vi "XBMC Send Input Action.vi"() -> ()   [LabVIEW 2013, in "LVH-XBMC.lvlib"]
doc: "This example demonstrates how to send basic input actions to a local or remote XBMC instance."
uses:
  vi.lib/LabVIEW Hacker/XBMC/LVH-XBMC.lvlib
  vi.lib/LabVIEW Hacker/XBMC/Private/Type Defs/JSON_Objects/Input_Action.ctl
panel:
  in  "Port (80)":u16=80
  in  "Stop Button":bool
  in  "Select Button":bool
  in  "Back Button":bool
  in  "Right Button":bool
  in  "Left Button":bool
  in  "Down Button":bool
  in  "Up Button":bool
  in  "Hostname / IP":string="localhost"
  in  "Username":string
  in  "Password":string
  # "XBMC Basic Input Action Example\n\nThis example demonstrates how to send basic input actions to a local or remote XBMC instance.\n\n1. Enter the Hostname or IP Address of the XBMC instance you want to control.\n     Note: The XBMC webserver must be enabled for the LabVIEW XBMC API to work. \n2. Enter the Username and Password you've assigned to the XBMC instance.\n3. Click the Run Arrow.\n4. Click the buttons on this LabVIEW front panel to send input actions to the XBMC instance."
  # "Configure"
  # "Control"
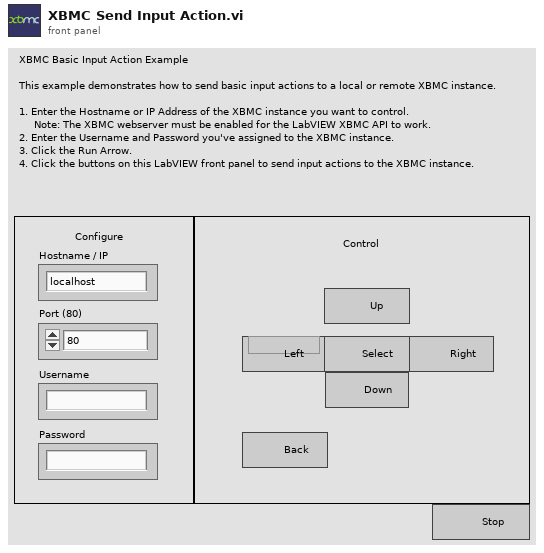
[diagram p1: front panel]
types:
  T1 = typedef "LVH-XBMC.lvlib/XBMC Ref.ctl" = cluster{"HTTP Handle":T2, "Hostname / IP":string, "jsonrpc":string}
  T2 = typedef "LabVIEWHTTPClient.lvlib/ClientHandle.ctl" = refnum<k1>
  T3 = typedef "LVH-XBMC.lvlib/Input_Action.ctl" = enum16{"left", "right", "up", "down", "pageup", "pagedown", "select", "highlight", "parentdir", "parentfolder", "back", "previousmenu", "info", "pause", "stop", "skipnext", "skipprevious", "fullscreen", "aspectratio", "stepforward", "stepback", "bigstepforward", "bigstepback", "chapterorbigstepforward", "chapterorbigstepback", "osd", "showsubtitles", "nextsubtitle", "codecinfo", "nextpicture", "previouspicture", "zoomout", "zoomin", "playlist", "queue", "zoomnormal", "zoomlevel1", "zoomlevel2", "zoomlevel3", "zoomlevel4", "zoomlevel5", "zoomlevel6", "zoomlevel7", "zoomlevel8", "zoomlevel9", "nextcalibration", "resetcalibration", "analogmove", "rotate", "rotateccw", "close", "subtitledelayminus", "subtitledelay", "subtitledelayplus", "audiodelayminus", "audiodelay", "audiodelayplus", "subtitleshiftup", "subtitleshiftdown", "subtitlealign", "audionextlanguage", "verticalshiftup", "verticalshiftdown", "nextresolution", "audiotoggledigital", "number0", "number1", "number2", "number3", "number4", "number5", "number6", "number7", "number8", "number9", "osdleft", "osdright", "osdup", "osddown", "osdselect", "osdvalueplus", "osdvalueminus", "smallstepback", "fastforward", "rewind", "play", "playpause", "switchplayer", "delete", "copy", "move", "mplayerosd", "hidesubmenu", "screenshot", "rename", "togglewatched", "scanitem", "reloadkeymaps", "volumeup", "volumedown", "mute", "backspace", "scrollup", "scrolldown", "analogfastforward", "analogrewind", "moveitemup", "moveitemdown", "contextmenu", "shift", "symbols", "cursorleft", "cursorright", "showtime", "analogseekforward", "analogseekback", "showpreset", "presetlist", "nextpreset", "previouspreset", "lockpreset", "randompreset", "increasevisrating", "decreasevisrating", "showvideomenu", "enter", "increaserating", "decreaserating", "togglefullscreen", "nextscene", "previousscene", "nextletter", "prevletter", "jumpsms2", "jumpsms3", "jumpsms4", "jumpsms5", "jumpsms6", "jumpsms7", "jumpsms8", "jumpsms9", "filter", "filterclear", "filtersms2", "filtersms3", "filtersms4", "filtersms5", "filtersms6", "filtersms7", "filtersms8", "filtersms9", "firstpage", "lastpage", "guiprofile", "red", "green", "yellow", "blue", "increasepar", "decreasepar", "volampup", "volampdown", "createbookmark", "createepisodebookmark", "settingsreset", "settingslevelchange", "stereomode", "nextstereomode", "previousstereomode", "togglestereomode", "stereomodetomono", "channelup", "channeldown", "previouschannelgroup", "nextchannelgroup", "playpvr", "playpvrtv", "playpvrradio", "record", "leftclick", "rightclick", "middleclick", "doubleclick", "wheelup", "wheeldown", "mousedrag", "mousemove", "tap", "longpress", "pangesture", "zoomgesture", "rotategesture", "swipeleft", "swiperight", "swipeup", "swipedown", "noop"}
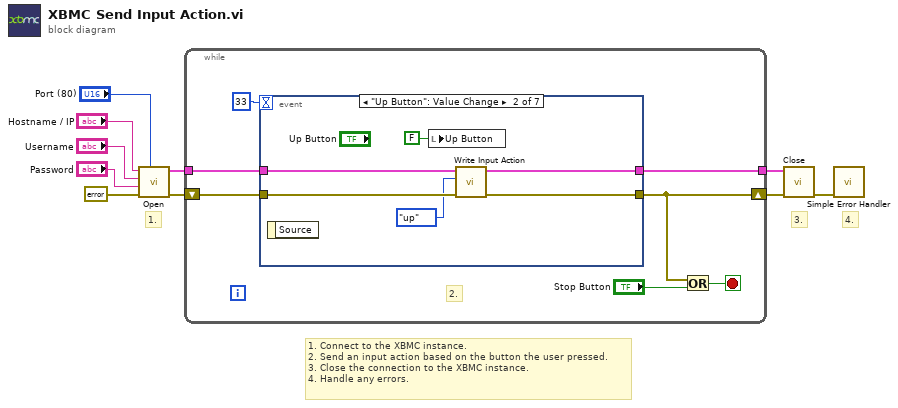
[diagram p0: block diagram]
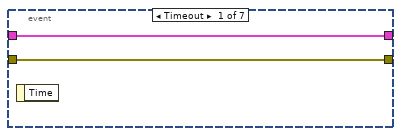
[diagram p2: hidden frame]
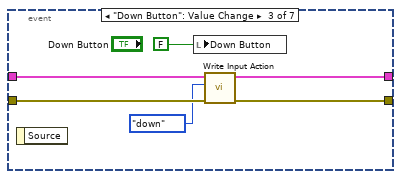
[diagram p3: hidden frame]
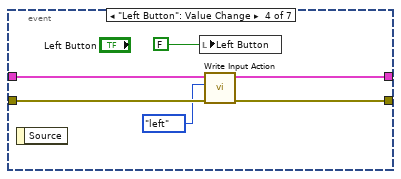
[diagram p4: hidden frame]
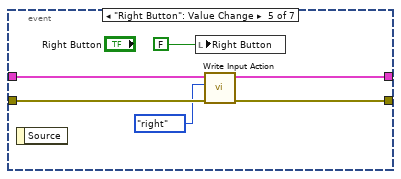
[diagram p5: hidden frame]
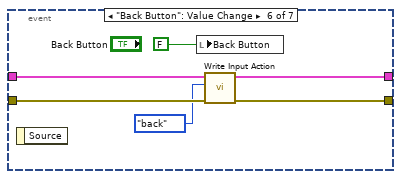
[diagram p6: hidden frame]
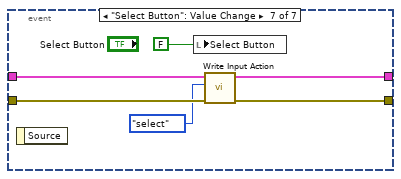
[diagram p7: hidden frame]
diagram:
  # "1. Connect to the XBMC instance.\n2. Send an input action based on the button the user pressed.\n3. Close the connection to the XBMC instance.\n4. Handle any errors."
  # "4."
  # "3."
  # "1."
  n1 = call "Open.vi"("Port (80)"="Port (80)", "Error In"=errorcluster {"status"=FALSE, "code"=0, "source"=""}, "Password"="Password", "Username"="Username", "Hostname / IP"="Hostname / IP") -> ("Error Out"=w9:errorcluster, "XBMC Ref"=w10:T1)  [unwired: 5 in]
  n2 = while {
    tunnel: w10 -> [w17]
    tunnel: [w15] -> w4
    shift-right: [w12] -> w3
    shift-left: w9 -> [w16]
    stop <- w14 stop-if-true
    # "2."
    n3 = event shown="[1] \"Up Button\": Value Change" {
      selector: _ -> [_ _ _ _ _ _ _]
      dyn-events: _ -> [_ _ _ _ _ _ _]
      timeout: 33 -> [_ _ _ _ _ _ _]
      tunnel: w17 -> [w19 w22 w28 w34 w40 w46 w52]
      tunnel: w16 -> [w18 w21 w27 w33 w39 w45 w51]
      tunnel: [w19 w24 w30 w36 w42 w48 w54] -> w15
      tunnel: [w18 w23 w29 w35 w41 w47 w53] -> w12
      event Timeout {
        n4 = event-data() -> ()  [unwired: 1 in, 1 out]
      }
      event "Up Button": Value Change {
        n5 = event-data() -> ()  [unwired: 1 in, 1 out]
        n6 = local write "Up Button"(FALSE ("Up Button")) -> ()
        n7 = call "Write Input Action.vi"("Error In"=w21, "Input Action"=Input_Action."up", "XBMC Ref"=w22) -> ("Error Out"=w23:errorcluster, "XBMC Ref"=w24:T1)  [unwired: 7 in]
      }
      event "Down Button": Value Change {
        n8 = event-data() -> ()  [unwired: 1 in, 1 out]
        n9 = local write "Down Button"(FALSE ("Up Button")) -> ()
        n10 = call "Write Input Action.vi"("Error In"=w27, "Input Action"=Input_Action."down", "XBMC Ref"=w28) -> ("Error Out"=w29:errorcluster, "XBMC Ref"=w30:T1)  [unwired: 7 in]
      }
      event "Left Button": Value Change {
        n11 = event-data() -> ()  [unwired: 1 in, 1 out]
        n12 = local write "Left Button"(FALSE ("Up Button")) -> ()
        n13 = call "Write Input Action.vi"("Error In"=w33, "Input Action"=Input_Action."left", "XBMC Ref"=w34) -> ("Error Out"=w35:errorcluster, "XBMC Ref"=w36:T1)  [unwired: 7 in]
      }
      event "Right Button": Value Change {
        n14 = event-data() -> ()  [unwired: 1 in, 1 out]
        n15 = local write "Right Button"(FALSE ("Up Button")) -> ()
        n16 = call "Write Input Action.vi"("Error In"=w39, "Input Action"=Input_Action."right", "XBMC Ref"=w40) -> ("Error Out"=w41:errorcluster, "XBMC Ref"=w42:T1)  [unwired: 7 in]
      }
      event "Back Button": Value Change {
        n17 = event-data() -> ()  [unwired: 1 in, 1 out]
        n18 = local write "Back Button"(FALSE ("Up Button")) -> ()
        n19 = call "Write Input Action.vi"("Error In"=w45, "Input Action"=Input_Action."back", "XBMC Ref"=w46) -> ("Error Out"=w47:errorcluster, "XBMC Ref"=w48:T1)  [unwired: 7 in]
      }
      event "Select Button": Value Change {
        n20 = event-data() -> ()  [unwired: 1 in, 1 out]
        n21 = local write "Select Button"(FALSE ("Up Button")) -> ()
        n22 = call "Write Input Action.vi"("Error In"=w51, "Input Action"=Input_Action."select", "XBMC Ref"=w52) -> ("Error Out"=w53:errorcluster, "XBMC Ref"=w54:T1)  [unwired: 7 in]
      }
    }
    n23 = Or(x=w12, y="Stop Button") -> (x .or. y?=w14:bool)
  }
  n24 = call "Close.vi"("Error In"=w3, "XBMC Ref"=w4) -> ("Error Out"=w2:errorcluster)  [unwired: 9 in]
  n25 = call <vilib>:"Simple Error Handler.vi"("error in (no error)"=w2) -> ()  [unwired: 4 in, 5 out]
